vi "get image 2.vi"() -> ()   [LabVIEW 2012]
uses:
  <vilib>/vision/driver/NI_Vision_Acquisition_Software.lvlib
  <vilib>/userdefined/High Color/IMAQdx.ctl
panel:
  in  "Stop Button":bool
  in  "Session In":T1
  out "Image":T2(plugin-control)
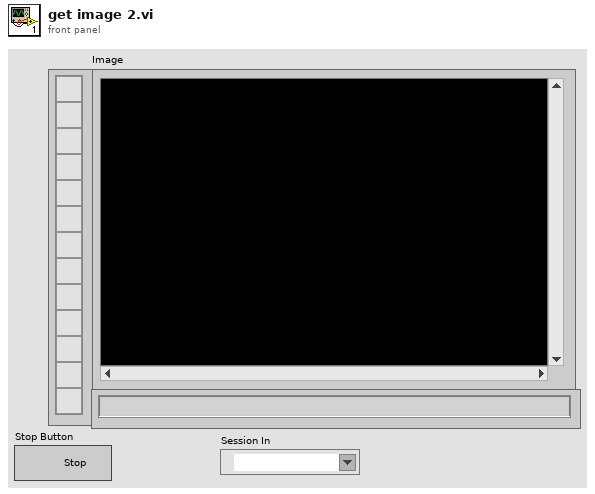
[diagram p1: front panel]
types:
  T1 = typedef "IMAQdx.ctl" = refnum<k21>
  T2 = typedef "IMAQ Image.ctl" = refnum<image>
  T3 = typedef "Image Type" = u32
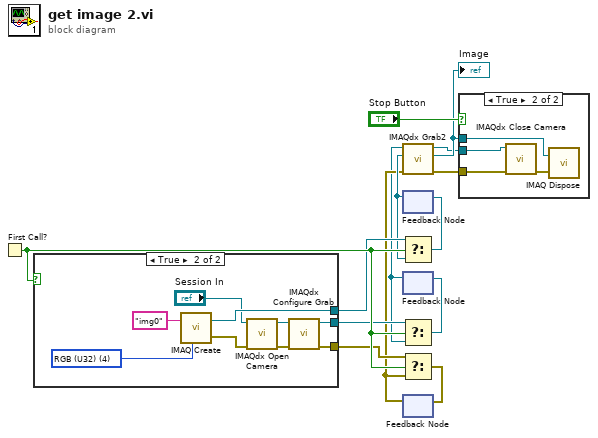
[diagram p0: block diagram]
diagram:
  n1 = First Call?() -> (First Call?: T/F=w8:bool)
  n2 = case shown="True" w8 {
    tunnel: [_ w20] -> w7
    tunnel: [_ w19] -> w6
    tunnel: [_ w18] -> w5
    frame False {
    }
    frame True {
      w17 = T3 4 items=["Grayscale (U8)", "Grayscale (I16)", "Grayscale (SGL)", "Complex (CSG)", "RGB (U32)", "HSL (U32)", "RGB (U64)", "Grayscale (U16)"] ("Image Type")
      n3 = call "IMAQ Create"("Image Name"="img0", "Image Type"=w17) -> ("New Image"=w20:T2, "error out"=w23:errorcluster)  [unwired: 3 in]
      n4 = call <vilib>:"IMAQdx Open Camera.vi"("error in"=w23, "Session In"="Session In") -> ("error out"=w21:errorcluster, "Session Out"=w22:T1)  [unwired: 8 in]
      n5 = call <vilib>:"IMAQdx Configure Grab.vi"("error in"=w21, "Session In"=w22) -> ("error out"=w18:errorcluster, "Session Out"=w19:T1)  [unwired: 8 in]
    }
  }
  n6 = feedback #1() -> (w4:T2)  [unwired: 1 in]
  n7 = Select(t=w7, s=w8, f=w4) -> (s? t:f=w10:T2)
  n8 = feedback-in #1(w10) -> ()
  n9 = feedback #2() -> (w1:T1)  [unwired: 1 in]
  n10 = Select(t=w6, s=w8, f=w1) -> (s? t:f=w3:T1)
  n11 = feedback-in #2(w3) -> ()
  n12 = feedback #3() -> (w2:errorcluster)  [unwired: 1 in]
  n13 = call <vilib>:"IMAQdx Grab2.vi"("error in"=w2, "Image In"=w4, "Session In"=w1) -> ("error out"=w12:errorcluster, "Image Out"=w13:T2, "Session Out"=w11:T1)  [unwired: 5 in, 1 out]
  "Image" <- w13
  n14 = Select(t=w5, s=w8, f=w2) -> (s? t:f=w9:errorcluster)
  n15 = feedback-in #3(w9) -> ()
  n16 = case shown="True" "Stop Button" {
    tunnel: w13 -> [_ w26]
    tunnel: w11 -> [_ w25]
    tunnel: w12 -> [_ w24]
    frame False {
    }
    frame True {
      n17 = call <vilib>:"IMAQdx Close Camera.vi"("error in"=w24, "Session In"=w25) -> ("error out"=w27:errorcluster)  [unwired: 9 in]
      n18 = call "IMAQ Dispose"("Image"=w26, "error in (no error)"=w27) -> ()  [unwired: 4 in, 1 out]
    }
  }
